vi "Write Global Locked.vi"(8 "error in (no error)":errorcluster, 10 "Global":refnum<class "System.lvclass">, 11 "GrabberWheels in":refnum<class "GrabberWheels.lvclass">) -> (0 "error out":errorcluster, 3 "GrabberWheels out":refnum<class "GrabberWheels.lvclass">)   [LabVIEW 2013, in "GrabberWheels.lvclass"]
uses:
  GrabberWheels.lvclass
  System/System.lvclass
  Robot Global Data.vi
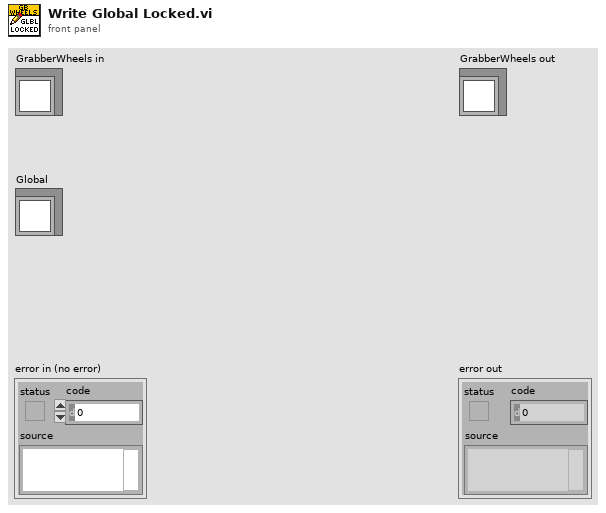
[diagram p1: front panel]
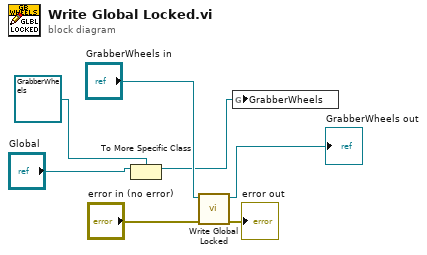
[diagram p0: block diagram]
diagram:
  n1 = To More Specific Class(target class=refnum<class "GrabberWheels.lvclass"> refnum ("GrabberWheels.lvclass"), reference="Global") -> (specific class reference=w1:refnum<class "GrabberWheels.lvclass">)  [unwired: 1 in, 1 out]
  n2 = call-parent "Write Global Locked.vi"("error in (no error)"="error in (no error)", "System in"="GrabberWheels in") -> ("error out"=→"error out":errorcluster, "System out"=→"GrabberWheels out":refnum<class "GrabberWheels.lvclass">)  [unwired: 8 in]
  n3 = global write "Robot Global Data.vi" "GrabberWheels"(w1) -> ()
